vi "Update Status Message for Test.vi"(11 "RF PostFlash in":refnum<class "RF PostFlash.lvclass">) -> ()   [LabVIEW 2015, in "RF PostFlash.lvclass"]
uses:
  RF PostFlash.lvclass
  Test Class/Test Class.lvclass
  Classes/Application/Class/Application.lvclass
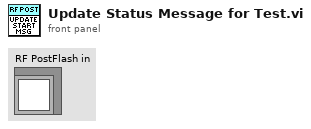
[diagram p1: front panel]
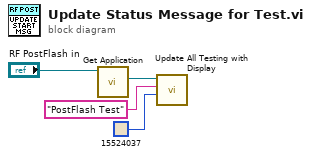
[diagram p0: block diagram]
diagram:
  n1 = call "Get Application.vi"("Test Class in"="RF PostFlash in") -> ("Application.lvlib:Application.lvclass"=w2:refnum<class "Application.lvclass">)  [unwired: 9 in, 1 out]
  n2 = call "Update All Testing with Display.vi"("BG Color"=u32 15524037, "Message ('')"="PostFlash Test", "Application in"=w2) -> ()  [unwired: 7 in, 2 out]
